vi "S-Curve Goal to Velocity2.vi"(8 "t":dbl, 9 "j":dbl, 10 "a":dbl, 11 "goal":dbl) -> (3 "v":dbl)   [LabVIEW 2020]
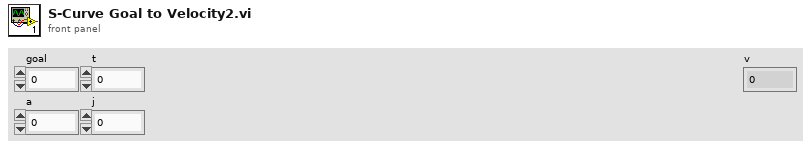
[diagram p1: front panel]
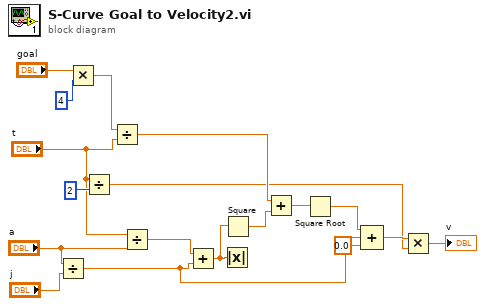
[diagram p0: block diagram]
diagram:
  n1 = Divide(x="a", y="j") -> (x/y=w3:dbl)
  n2 = Multiply(x="goal", y=4) -> (x*y=w13:dbl)
  n3 = Divide(x="t", y=2) -> (x/y=w5:dbl)
  n4 = Divide(x=w13, y="t") -> (x/y=w9:dbl)
  n5 = Divide(x="t", y="a") -> (x/y=w2:dbl)
  n6 = Add(x=w2, y=w3) -> (x+y=w11:dbl)
  n7 = Absolute Value(x=w11) -> ()  [unwired: 1 out]
  n8 = Square(x=w11) -> (x^2=w10:dbl)
  n9 = Add(x=w9, y=w10) -> (x+y=w8:dbl)
  n10 = Square Root(x=w8) -> (sqrt(x)=w7:dbl)
  n11 = Compound Arithmetic op=ADD(w7, w3, 0.0 ("value")) -> (w6:dbl)
  n12 = Multiply(x=w6, y=w5) -> (x*y=→"v":dbl)
